vi "NTV_AutoSelected String.vi"(7 "Read(f) Write(t)":bool, 11 "Auto Selected":string) -> (3 "Auto Selected":string)   [LabVIEW 2023]
uses:
  <vilib>/Rock Robotics/Network Tables/NT Read String.vi
  <vilib>/Rock Robotics/Network Tables/NT Write String.vi
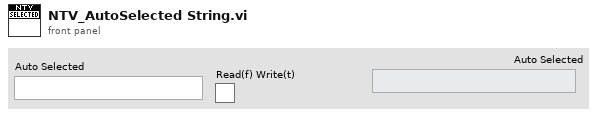
[diagram p1: front panel]
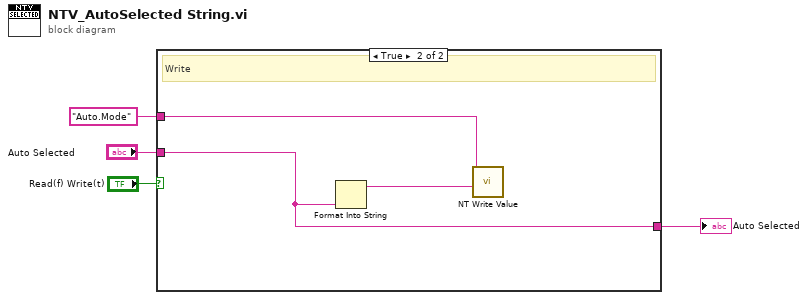
[diagram p0: block diagram]
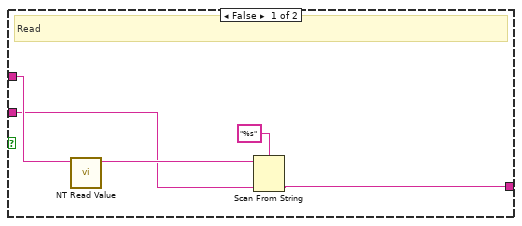
[diagram p2: hidden frame]
diagram:
  n1 = case shown="True" "Read(f) Write(t)" {
    tunnel: "Auto.Mode" ("Name") -> [w7 w12]
    tunnel: [w6 w10] -> w2
    tunnel: "Auto Selected" -> [w5 w10]
    frame False {
      # "Read"
      n2 = call-poly <vilib>:"NT Read Value.vi"("name"=w7) -> ("value"=w8:string)  [unwired: 8 in, 2 out]
      n3 = Scan From String(format string="%s", input string=w8, default 1=w5) -> (output 1=w6:string)  [unwired: 2 in, 3 out]
    }
    frame True {
      # "Write"
      n4 = Format Into String(w10) -> (resulting string=w11:string)  [unwired: 3 in, 1 out]
      n5 = call-poly <vilib>:"NT Write Value.vi"("value"=w11, "name"=w12) -> ()  [unwired: 9 in, 1 out]
    }
  }
  "Auto Selected" <- w2
